vi "OEE_PULSE_check_for_error.vi"(8 "OEE_PULSE_loop_state_in":T1, 11 "error_in":errorcluster) -> (0 "OEE_PULSE_loop_state_out":T1, 3 "error_out":errorcluster)   [LabVIEW 2019]
uses:
  OEE_PULSE_sequence_state.ctl
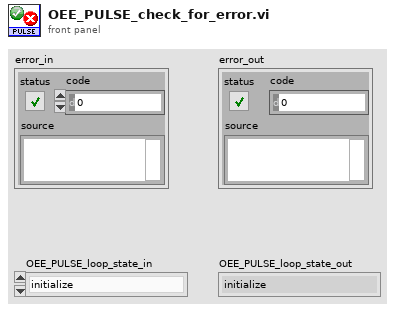
[diagram p1: front panel]
types:
  T1 = typedef "OEE_PULSE_sequence_state.ctl" = enum16{"initialize", "get_next_state", "start_pulses", "stop_pulses", "pulse", "error", "stop"}
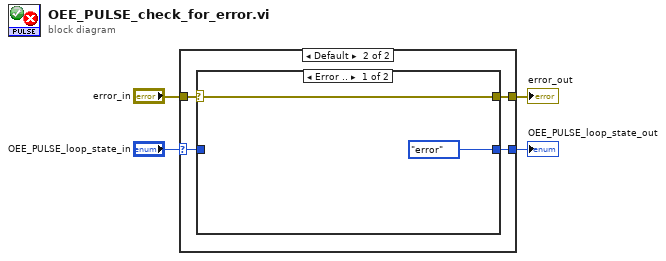
[diagram p0: block diagram]
diagram:
  n1 = case shown="Default" "OEE_PULSE_loop_state_in" {
    selector: "OEE_PULSE_loop_state_in" -> [w6 w8]
    tunnel: [w5 w10] -> w4
    tunnel: [w6 w9] -> w3
    tunnel: "error_in" -> [w5 w7]
    frame "stop" {
    }
    frame Default {
      n2 = case shown="Error .." w7 {
        selector: w7 -> [w12 w13]
        tunnel: [OEE_PULSE_sequence_state."error" ("OEE_PULSE_loop_state_in") w14] -> w9
        tunnel: w8 -> [_ w14]
        tunnel: [w12 w13] -> w10
        frame Error {
        }
        frame No Error {
        }
      }
    }
  }
  "error_out" <- w4
  "OEE_PULSE_loop_state_out" <- w3
